vi "Get From List.vi"(8 "error in (no error)":errorcluster caption="错误输入（无错误）", 11 "List 输入":refnum<class "List.lvclass"> caption="DNL_LabVIEW Object in") -> (0 "error out":errorcluster caption="错误输出", 2 "List.lvlib:DATA.lvclass":refnum<class "DATA.lvclass">, 3 "List 输出":refnum<class "List.lvclass"> caption="DNL_LabVIEW Object out")   [LabVIEW 2011, in "List.lvlib" / "List.lvclass"]
uses:
  List.lvclass
  data/DATA.lvclass
  List.lvclass/List.ctl
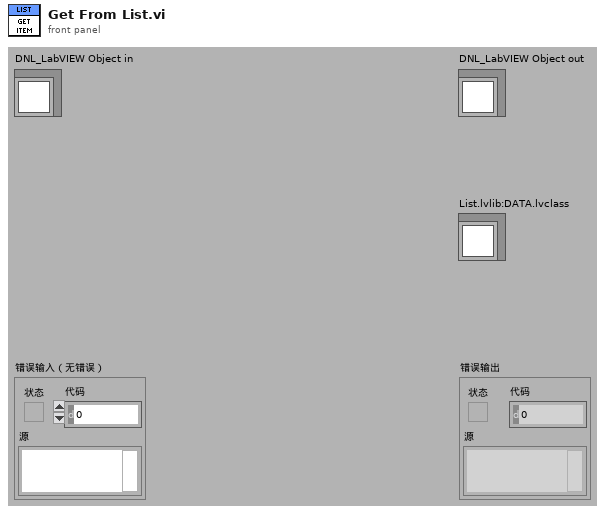
[diagram p1: front panel]
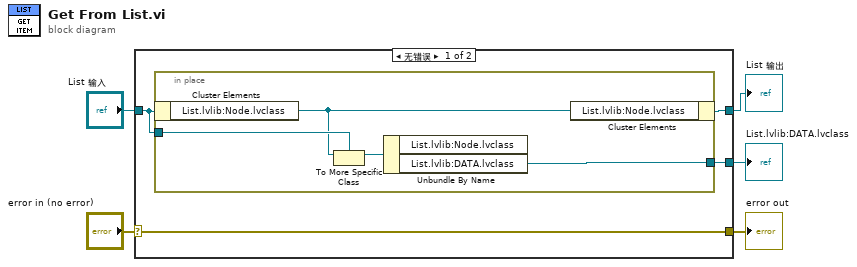
[diagram p0: block diagram]
diagram:
  n1 = case shown="无错误" "error in (no error)" {
    selector: "error in (no error)" -> [w9 w15]
    tunnel: [w9 w15] -> w4
    tunnel: [w6 w14] -> w2
    tunnel: "List 输入" -> [w8 w14]
    tunnel: [w7 _] -> w1
    frame No Error {
      n2 = in-place {
        in-place-border: w8 -> [w13]
        in-place-border: [w11] -> w7
        n3 = in-place-cluster #1(w8) -> ("List.lvlib:Node.lvclass"=w10:refnum<class "Node.lvclass">)
        n4 = To More Specific Class(target class=w13, reference=w10) -> (specific class reference=w12:refnum<class "List.lvclass">)  [unwired: 1 in, 1 out]
        n5 = Unbundle By Name(w12) -> ("List.lvlib:DATA.lvclass"=w11:refnum<class "DATA.lvclass">)  [unwired: 1 out]
        n6 = in-place-cluster #1("List.lvlib:Node.lvclass"=w10) -> (w6:refnum<class "List.lvclass">)
      }
    }
    frame Error {
    }
  }
  "error out" <- w4
  "List 输出" <- w2
  "List.lvlib:DATA.lvclass" <- w1
